vi "ATF Storage-AI V Start.vi"(8 "error in":errorcluster, 9 "AI V":T1(array[cluster]), 11 "Refnum in":refnum<k21>) -> (0 "error out":errorcluster, 3 "Refnum out":refnum<k21>)   [LabVIEW 2022 SP3]
doc: "This VI is for start for Analog voltage Start task"
uses:
  <vilib>/DAQmx/configure/timing.llb/DAQmx Timing (Sample Clock).vi
  <vilib>/DAQmx/configure/trigger.llb/DAQmx Start Trigger (Time).vi
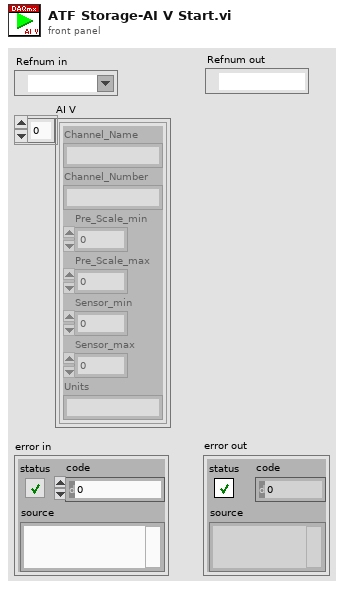
[diagram p1: front panel]
types:
  T1 = cluster{"Channel_Name":string, "Channel_Number":string, "Pre_Scale_min":dbl, "Pre_Scale_max":dbl, "Sensor_min":dbl, "Sensor_max":dbl, "Units":string}[]
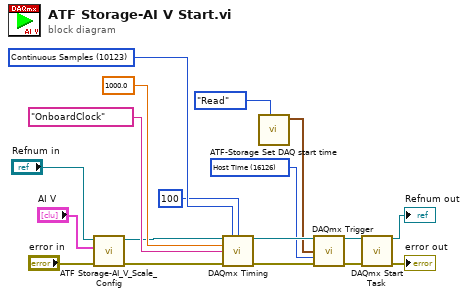
[diagram p0: block diagram]
diagram:
  w3 = 16126 items=["Host Time"=16126, "I/O Device Time"=16127] ("timescale")
  w12 = 10123 items=["Finite Samples"=10178, "Continuous Samples"=10123, "Hardware Timed Single Point"=12522] ("sample mode")
  n1 = call "ATF Storage-AI_V_Scale_Config.vi"("error in"="error in", "AI C"="AI V", "task in"="Refnum in") -> ("error out"=w5:errorcluster, "task out"=w10:refnum<k21>)  [unwired: 7 in]
  n2 = call-poly <vilib>:"DAQmx Timing.vi"("task/channels in"=w10, "sample mode"=w12, "samples per channel"=100, "rate"=1000.0, "source"=tag "OnboardClock", "error in"=w5) -> ("task out"=w15:refnum<k21>, "error out"=w8:errorcluster)  [unwired: 8 in]
  n3 = call "ATF-Storage Set DAQ start time.vi"("Enum"=enum16{"Read", "Write"}."Read") -> ("Start time 2"=w1:timestamp)  [unwired: 10 in]
  n4 = call-poly <vilib>:"DAQmx Trigger.vi"("task/channels in"=w15, "when"=w1, "timescale"=w3, "error in"=w8) -> ("task out"=w17:refnum<k21>, "error out"=w16:errorcluster)  [unwired: 10 in]
  n5 = call <vilib>:"DAQmx Start Task.vi"("task/channels in"=w17, "error in"=w16) -> ("task out"=→"Refnum out":refnum<k21>, "error out"=→"error out":errorcluster)  [unwired: 12 in]
